vi "SVD_Probe.vi"(11 "SVD":refnum<class "SVD.lvclass">) -> (2 "Value String":string, 3 "Pause VI":bool)   [LabVIEW 2020, in "OpenLvVision_OpenCv.lvlib" / "SVD.lvclass"]
uses:
  SVD.lvclass
  C:/Users/lukas/Downloads/OpenLvVision_OpenCv/SourceCode/LabView/OpenLvVision_OpenCv/_LvHelpers/EdvrObject/EdvrObject.lvclass
  _LvHelpers/EdvrObject/EdvrObject.lvclass/EdvrObject.ctl
  _LvHelpers/MatHandling/WriteSize/WriteSizeMat.vi
  _LvHelpers/MatHandling/WriteSize/WriteSizeMat_2DArray_SGL.vi
  _LvHelpers/MatHandling/RegisterMat/RegisterMat_Dll.vi
  _LvHelpers/MatHandling/RegisterMat/RegisterMat_Array2D-SGL.vi
  <vilib>/Utility/error.llb/Error Cluster From Error Code.vi
  _LvHelpers/MatHandling/UnregisterMat/UnregisterMat_Dll.vi
  _LvHelpers/MatHandling/UnregisterMat/UnregisterMat_2DArray-SGL.vi
  _LvHelpers/MatHandling/WriteSize/WriteSizeMat_2DArray_DBL.vi
  _LvHelpers/MatHandling/RegisterMat/RegisterMat_Array2D-DBL.vi
  _LvHelpers/MatHandling/UnregisterMat/UnregisterMat_2DArray-DBL.vi
  _LvHelpers/EdvrObject/EdvrObject.lvclass
panel:
  in  "Tab Control":enum32{"U", "VT", "W"}(tab)
  out "U":dbl[][](array[numeric])
  out "VT":dbl[][](array[numeric])
  out "W":dbl[][](array[numeric])
  out "Reference":u64 format="%.0x"
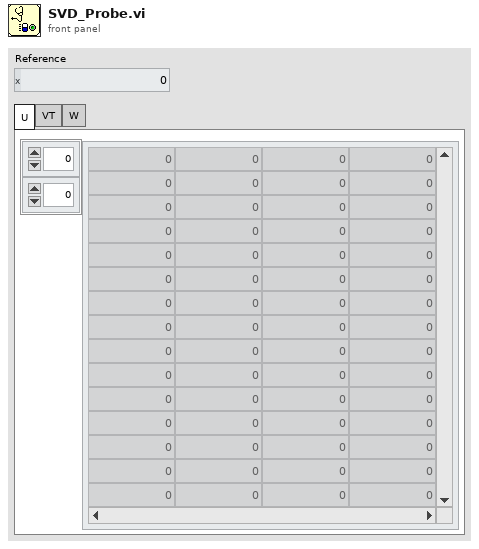
[diagram p1: front panel]
types:
  T1 = typedef "OpenLvVision_OpenCv.lvlib/EdvrObject.lvclass/Edvr.ctl" = refnum<data-value>
  T2 = typedef "OpenLvVision_OpenCv.lvlib/LvDatatype.ctl" = enum32{"Undefined", "U8", "I8", "U16", "I16", "U32_Color", "I32", "U64_Color", "I64", "SGL", "DBL", "Complex SGL", "Complex DBL", "Array 1D U8", "Array 1D I8", "Array 1D U16", "Array 1D I16", "Array 1D U32_Color", "Array 1D I32", "Array 1D U64_Color", "Array 1D I64", "Array 1D SGL", "Array 1D DBL", "Array 1D Complex SGL", "Array 1D Complex DBL", "Array 2D U8", "Array 2D I8", "Array 2D U16", "Array 2D I16", "Array 2D U32", "Array 2D U32_Color", "Array 2D I32", "Array 2D U64", "Array 2D U64_Color", "Array 2D I64", "Array 2D SGL", "Array 2D DBL", "Array 2D Complex SGL", "Array 2D Complex DBL", "Image Mono U8", "Image Mono U16", "Image Mono I16", "Image Mono SGL", "Image Color U32", "Image Color U64", "ImageComplex Sgl", "Array1d_2dPointI32", "Array1d_2dPointSGL", "Array1d_2dPointDBL", "Array1d_3dPointI32", "Array1d_3dPointSGL", "Array1d_3dPointDBL", "Array1d_4dPointI32", "Array1d_4dPointSGL", "Array1d_4dPointDBL"}
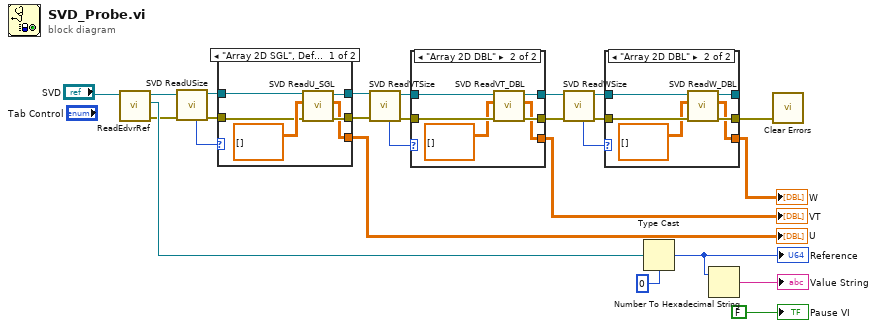
[diagram p0: block diagram]
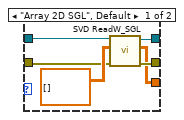
[diagram p2: hidden frame]
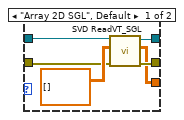
[diagram p3: hidden frame]
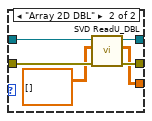
[diagram p4: hidden frame]
diagram:
  n1 = call "ReadEdvrRef.vi"("EdvrObject in"="SVD") -> ("error out"=w18:errorcluster, "Edvr"=w23:T1, "EdvrObject out"=w19:refnum<class "SVD.lvclass">)  [unwired: 8 in]
  n2 = call "SVD ReadUSize.vi"("error in (no error)"=w18, "SVD in"=w19) -> ("error out"=w11:errorcluster, "SVD out"=w12:refnum<class "SVD.lvclass">, "Datatype"=w13:T2)  [unwired: 5 in, 2 out]
  n3 = case shown="\"Array 2D SGL\", Default" w13 {
    tunnel: w12 -> [w30 w37]
    tunnel: w11 -> [w29 w36]
    tunnel: [w28 w35] -> w9
    tunnel: [w27 w34] -> w10
    tunnel: [w26 w32] -> w17
    frame "Array 2D SGL", Default {
      n4 = call "SVD ReadU_SGL.vi"("error in (no error)"=w29, "Dst in"=sgl[][] [] ("W"), "SVD in"=w30) -> ("error out"=w28:errorcluster, "Dst  out"=w26:sgl[][], "SVD out"=w27:refnum<class "SVD.lvclass">)  [unwired: 6 in]
    }
    frame "Array 2D DBL" {
      n5 = call "SVD ReadU_DBL.vi"("error in (no error)"=w36, "Dst in"=dbl[][] [] ("W"), "SVD in"=w37) -> ("error out"=w35:errorcluster, "Dst  out"=w32:dbl[][], "SVD out"=w34:refnum<class "SVD.lvclass">)  [unwired: 6 in]
    }
  }
  "U" <- w17
  n6 = call "SVD ReadVTSize.vi"("error in (no error)"=w9, "SVD in"=w10) -> ("error out"=w8:errorcluster, "SVD out"=w7:refnum<class "SVD.lvclass">, "Datatype"=w6:T2)  [unwired: 5 in, 2 out]
  n7 = case shown="\"Array 2D DBL\"" w6 {
    tunnel: w7 -> [w42 w49]
    tunnel: w8 -> [w41 w48]
    tunnel: [w40 w47] -> w1
    tunnel: [w39 w46] -> w2
    tunnel: [w38 w44] -> w15
    frame "Array 2D SGL", Default {
      n8 = call "SVD ReadVT_SGL.vi"("error in (no error)"=w41, "Dst in"=sgl[][] [] ("W"), "SVD in"=w42) -> ("error out"=w40:errorcluster, "Dst  out"=w38:sgl[][], "SVD out"=w39:refnum<class "SVD.lvclass">)  [unwired: 6 in]
    }
    frame "Array 2D DBL" {
      n9 = call "SVD ReadVT_DBL.vi"("error in (no error)"=w48, "Dst in"=dbl[][] [] ("W"), "SVD in"=w49) -> ("error out"=w47:errorcluster, "Dst  out"=w44:dbl[][], "SVD out"=w46:refnum<class "SVD.lvclass">)  [unwired: 6 in]
    }
  }
  "VT" <- w15
  n10 = call "SVD ReadWSize.vi"("error in (no error)"=w1, "SVD in"=w2) -> ("error out"=w3:errorcluster, "SVD out"=w4:refnum<class "SVD.lvclass">, "Datatype"=w5:T2)  [unwired: 5 in, 2 out]
  n11 = case shown="\"Array 2D DBL\"" w5 {
    tunnel: w4 -> [w54 w61]
    tunnel: w3 -> [w53 w60]
    tunnel: [w52 w59] -> w16
    tunnel: [w51 w58] -> _
    tunnel: [w50 w56] -> w14
    frame "Array 2D SGL", Default {
      n12 = call "SVD ReadW_SGL.vi"("error in (no error)"=w53, "Dst in"=sgl[][] [] ("W"), "SVD in"=w54) -> ("error out"=w52:errorcluster, "Dst  out"=w50:sgl[][], "SVD out"=w51:refnum<class "SVD.lvclass">)  [unwired: 6 in]
    }
    frame "Array 2D DBL" {
      n13 = call "SVD ReadW_DBL.vi"("error in (no error)"=w60, "Dst in"=dbl[][] [] ("W"), "SVD in"=w61) -> ("error out"=w59:errorcluster, "Dst  out"=w56:dbl[][], "SVD out"=w58:refnum<class "SVD.lvclass">)  [unwired: 6 in]
    }
  }
  "W" <- w14
  n14 = Type Cast(type=u64 0, x=w23) -> (*(type *) &x=w22:u64)
  "Reference" <- w22
  n15 = Number To Hexadecimal String(2:w22) -> (0:→"Value String":string)  [unwired: 1 in]
  n16 = call <vilib>:"Clear Errors.vi"("error in (no error)"=w16) -> ()  [unwired: 5 in, 2 out]
  "Pause VI" <- FALSE
